vi "Read Worktable.vi"(8 "error in":errorcluster, 11 "Gluing Procedure in":refnum<class "Gluing Procedure.lvclass">) -> (0 "error out":errorcluster, 2 "WorkTable out":refnum<class "WorkTable Class.lvclass">, 3 "Gluing Procedure out":refnum<class "Gluing Procedure.lvclass">)   [LabVIEW 2011, in "Gluing Procedure.lvclass"]
uses:
  Gluing Procedure.lvclass
  Shared Components/WorkTable Class/WorkTable Class.lvclass
  Gluing Procedure.lvclass/Gluing Procedure.ctl
  Shared Components/Gantry Class/Gantry Class.lvclass
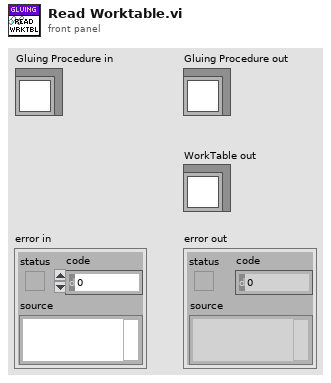
[diagram p1: front panel]
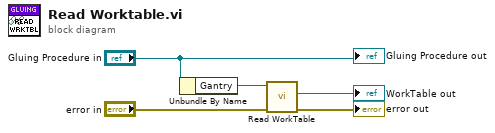
[diagram p0: block diagram]
diagram:
  n1 = Unbundle By Name("Gluing Procedure in") -> ("Gantry"=w3:refnum<class "Gantry Class.lvclass">)
  n2 = call-dynamic "Read WorkTable.vi"("error in"="error in", "Gantry Class in"=w3) -> ("error out"=→"error out":errorcluster, "WorkTable Class.lvclass"=→"WorkTable out":refnum<class "WorkTable Class.lvclass">)  [unwired: 7 in, 1 out]
  "Gluing Procedure out" <- "Gluing Procedure in"
